vi "LoadWithFood.vi"(1 "Input Array":i8[][](array[numeric]), 2 "Food Per Level":i32) -> (0 "Output Array":i8[][](array[numeric]))   [LabVIEW 2012]
doc: "Loads a 10x10 occupancy grid with N randomly placed food squares valued 1 to N."
panel:
  # "This VI places N food squares into the world, with one of each of the values from 1 to N:"
  # "food per level"
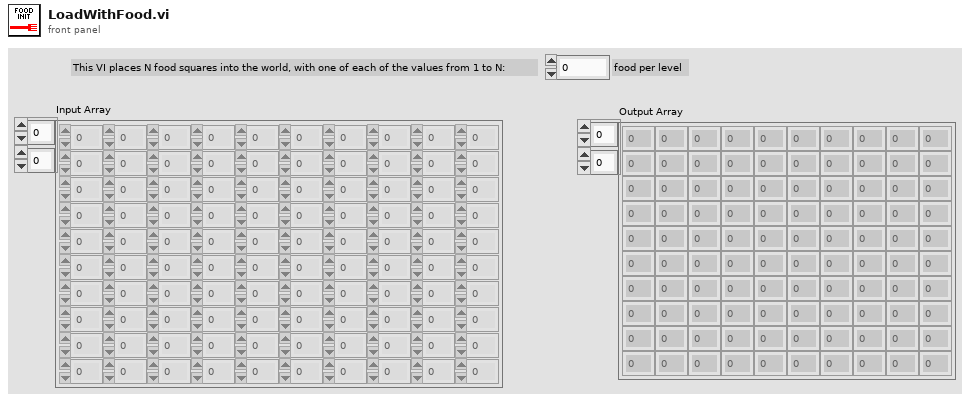
[diagram p1: front panel]
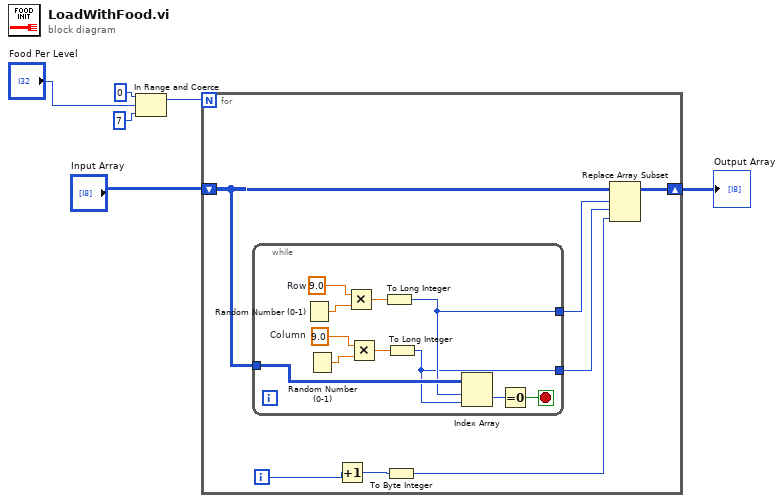
[diagram p0: block diagram]
diagram:
  n1 = In Range and Coerce(upper limit=0, x="Food Per Level", lower limit=7) -> (coerced(x)=w4:i32)  [unwired: 1 out]
  n2 = for {
    N: w4 -> [_]
    shift-right: [w13] -> w5
    shift-left: "Input Array" -> [w12]
    i -> [w9]
    n3 = while {
      tunnel: w12 -> [w23]
      tunnel: [w15] -> w11
      tunnel: [w14] -> w10
      stop <- w17 stop-if-true
      w19 = 9.0  # Column
      w22 = 9.0  # Row
      n4 = Random Number (0-1)() -> (number: 0 to 1=w21:dbl)
      n5 = Random Number (0-1)() -> (number: 0 to 1=w18:dbl)
      n6 = Multiply(x=w22, y=w21) -> (x*y=w24:dbl)
      n7 = Multiply(x=w19, y=w18) -> (x*y=w20:dbl)
      n8 = To Long Integer(number=w24) -> (32bit integer=w15:i32)
      n9 = To Long Integer(number=w20) -> (32bit integer=w14:i32)
      n10 = Index Array(array=w23, index (row)=w15, index (col)=w14) -> (element=w16:i8)
      n11 = Equal To 0?(x=w16) -> (x = 0?=w17:bool)
    }
    n12 = Increment(x=w9) -> (x+1=w8:i32)
    n13 = To Byte Integer(number=w8) -> (8bit integer=w7:i8)
    n14 = Replace Array Subset(array=w12, new element=w7, index (row)=w11, index (col)=w10) -> (w13:i8[][])
  }
  "Output Array" <- w5
